vi "CleanDefectiveCharIntoString.vi"(8 "error in (no error)":errorcluster, 10 "String In":string, 11 "object in":refnum<class "Crypter.lvclass">) -> (0 "error out":errorcluster, 2 "String Out":string, 3 "object out":refnum<class "Crypter.lvclass">)   [LabVIEW 2016, in "Crypter.lvclass"]
uses:
  Crypter.lvclass
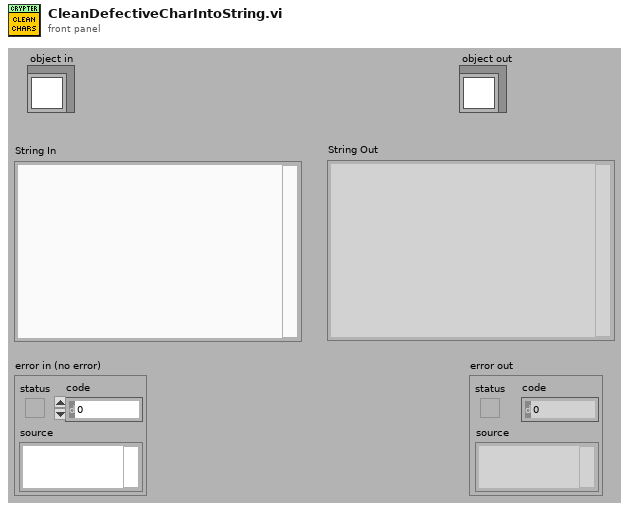
[diagram p1: front panel]
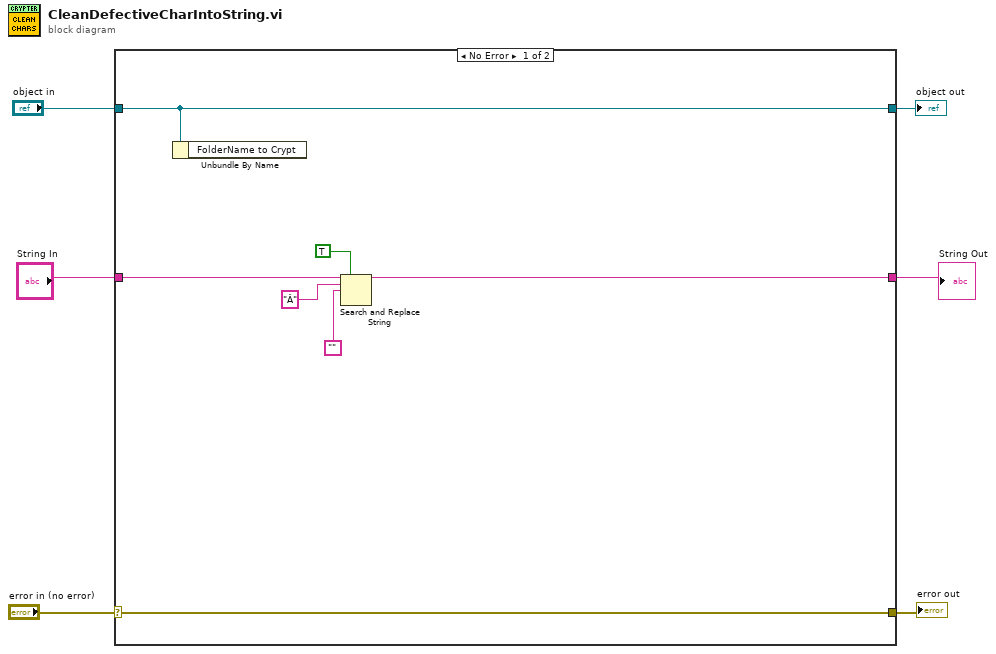
[diagram p0: block diagram]
diagram:
  n1 = case shown="No Error" "error in (no error)" {
    selector: "error in (no error)" -> [w13 w16]
    tunnel: [w13 w16] -> w5
    tunnel: [w12 w15] -> w3
    tunnel: "object in" -> [w12 w15]
    tunnel: "String In" -> [w11 w14]
    tunnel: [w10 w14] -> w1
    frame No Error {
      n2 = Unbundle By Name(w12) -> ()  [unwired: 1 out]
      n3 = Search and Replace String(replace all?=TRUE ("replace all? (F)"), input string=w11, search string="Â", replace string="") -> (result string=w10:string)  [unwired: 4 in, 3 out]
    }
    frame Error {
    }
  }
  "error out" <- w5
  "object out" <- w3
  "String Out" <- w1
